vi "BenchConstructor.vi"(11 "BenchModel":string) -> (0 "error out":errorcluster, 3 "BenchParent.lvclass":refnum<class "BenchParent.lvclass">)   [LabVIEW 2024]
uses:
  BenchParent.lvclass
  SmartBench/SmartBench.lvclass
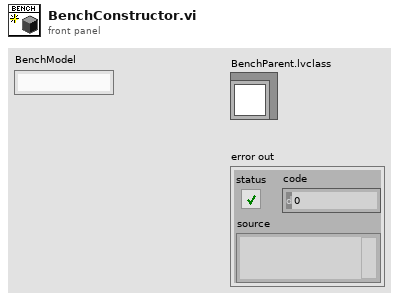
[diagram p1: front panel]
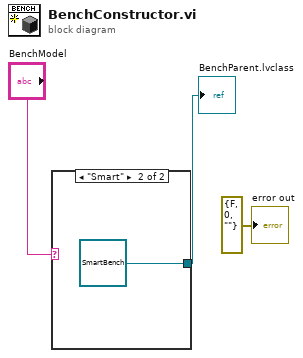
[diagram p0: block diagram]
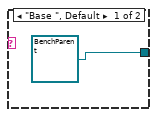
[diagram p2: hidden frame]
diagram:
  n1 = case shown="\"Smart\"" "BenchModel" {
    tunnel: [refnum<class "BenchParent.lvclass"> refnum ("BenchParent.lvclass") refnum<class "SmartBench.lvclass"> refnum ("SmartBench.lvclass")] -> w2
    frame "Base ", Default {
    }
    frame "Smart" {
    }
  }
  "BenchParent.lvclass" <- w2
  "error out" <- errorcluster {"status"=FALSE, "code"=0, "source"=""} ("error out")
